vi "Resideo Gas Valve Main.vi"(6 "Use Vesta Tool?":bool, 8 "error in (no error)":errorcluster, 11 "VISA resource name":refnum<visa-resource-name>) -> (0 "error out":errorcluster)   [LabVIEW 2023]
uses:
  Type Definitions/Temperature Control.ctl
  <vilib>/NI/Modbus Library/API/Wrapper/Create Serial Master.vi
  <vilib>/NI/Modbus Library/API/Master/Modbus Master.lvclass
  <vilib>/NI/Modbus Library/API/Wrapper/API Main.lvlib
panel:
  in  "Temperature Setpoint/Differential":T1 {"Water Heater Temp (°F)" min=32 max=203}
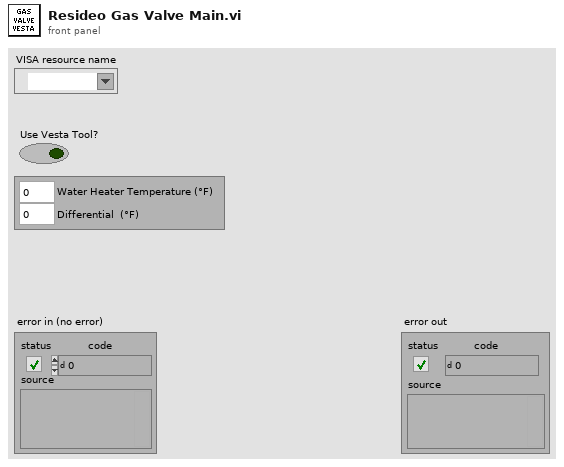
[diagram p1: front panel]
types:
  T1 = typedef "Temperature Control.ctl" = cluster{"Water Heater Temp (°F)":u16, "Differential  (°F)":dbl}
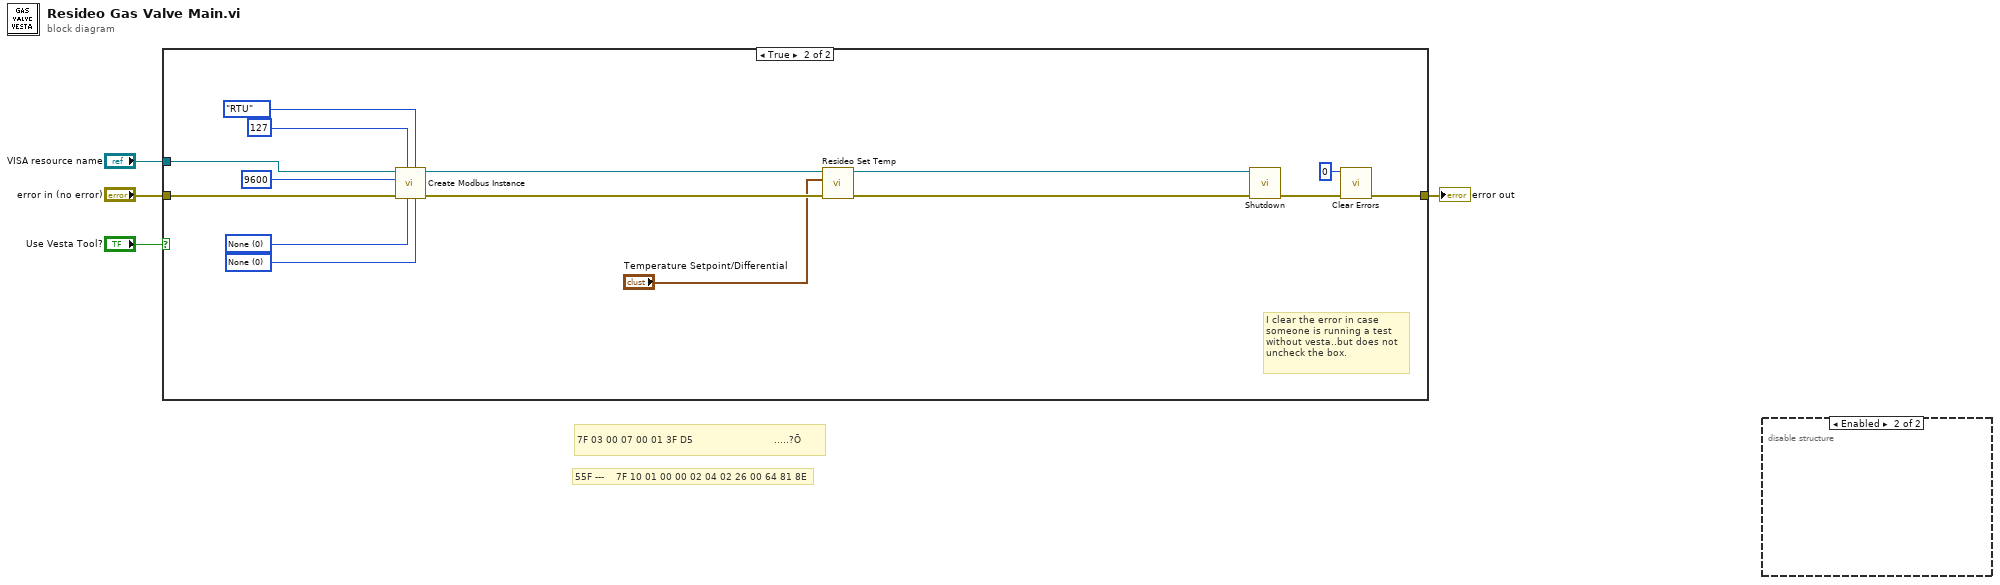
[diagram p0: block diagram]
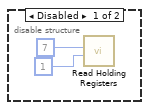
[diagram p3: hidden frame]
diagram:
  # "55F ---    7F 10 01 00 00 02 04 02 26 00 64 81 8E"
  # "7F 03 00 07 00 01 3F D5                           .....?Õ"
  n1 = case shown="True" "Use Vesta Tool?" {
    tunnel: "VISA resource name" -> [_ w20]
    tunnel: "error in (no error)" -> [w5 w14]
    tunnel: [w5 w8] -> w2
    frame False {
    }
    frame True {
      w15 = u16 0 items=["None", "XON/XOFF", "RTS/CTS", "XON/XOFF & RTS/CTS", "DTR/DSR", "XON/XOFF & DTR/DSR"] ("flow control (none)")
      w16 = u16 0 items=["None", "Odd", "Even", "Mark", "Space"] ("parity (even)")
      # "I clear the error in case\nsomeone is running a test\nwithout vesta..but does not\nuncheck the box."
      n2 = call-poly <vilib>:"Create Modbus Instance.vi"("flow control (none)"=w15, "serial type"=enum16{"RTU", "ASCII"}."RTU", "parity (even)"=w16, "unit ID"=u8 127, "error in"=w14, "baud rate"=u32 9600, "VISA resource name"=w20) -> ("error out"=w13:errorcluster, "serial master instance"=w11:refnum<class "Modbus Master.lvclass">)  [unwired: 3 in]
      n3 = call "Resideo Set Temp.vi"("error in (no error)"=w13, "Vesta Data"="Temperature Setpoint/Differential", "Modbus Master in"=w11) -> ("error out"=w12:errorcluster, "Modbus Master out"=w10:refnum<class "Modbus Master.lvclass">)  [unwired: 7 in]
      n4 = call-dynamic "Shutdown.vi"("error in"=w12, "Modbus master in"=w10) -> ("error out"=w9:errorcluster)  [unwired: 9 in]
      n5 = call <vilib>:"Clear Errors.vi"("error in (no error)"=w9, "specific error code to clear (0: all)"=0) -> ("error out"=w8:errorcluster)  [unwired: 4 in, 1 out]
    }
  }
  "error out" <- w2
  n6 = disable-structure shown="Enabled" {
    frame Disabled {
      n7 = call-dynamic "Read Holding Registers.vi"("number of inputs"=u16 1, "starting address"=u16 7) -> ()  [unwired: 7 in, 3 out]
    }
    frame Enabled {
    }
  }
